vi "readFromXML.vi"(8 "error in (no error)":errorcluster, 10 "XML in":string, 11 "WSSet in":refnum<class "WSSet.lvclass">) -> (0 "error out":errorcluster, 3 "WSSet out":refnum<class "WSSet.lvclass">)   [LabVIEW 2014, in "TCSDataDefinitions.lvlib" / "TCSWeatherServerCommand.lvlib" / "WSSet.lvclass"]
uses:
  WSSet.lvclass
  <userlib>/Common/UnitsAndXML/FlattenItemWithUnitToXML/FlattenPressureToXML/PressureUnit.ctl
  <userlib>/Common/UnitsAndXML/FlattenItemWithUnitToXML/FlattenTemperatureAbsToXML/TemperatureAbsUnit.ctl
  WSSet.lvclass/WSSet.ctl
  TCSWeatherServerCommand/TCSWeatherServerCommand.lvclass
  <userlib>/Common/UnitsAndXML/UnitsAndXML.lvlib
  <userlib>/Common/XML/XMLParser/XMLParser.lvclass
panel:
  out "relativeHumidity_percent":dbl
  out "temperature_degC":dbl[unit]=273.15
  out "pressure_mbar":dbl[unit]
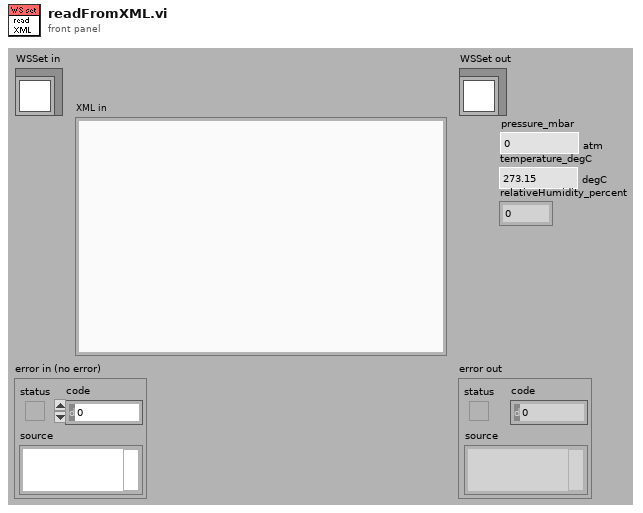
[diagram p1: front panel]
types:
  T1 = typedef "UnitsAndXML.lvlib/TemperatureAbsUnit.ctl" = enum16{"K", "degC", "degF"}
  T2 = typedef "UnitsAndXML.lvlib/PressureUnit.ctl" = enum16{"Pa", "atm", "bar", "mbar", "m.Hg", "psi", "torr"}
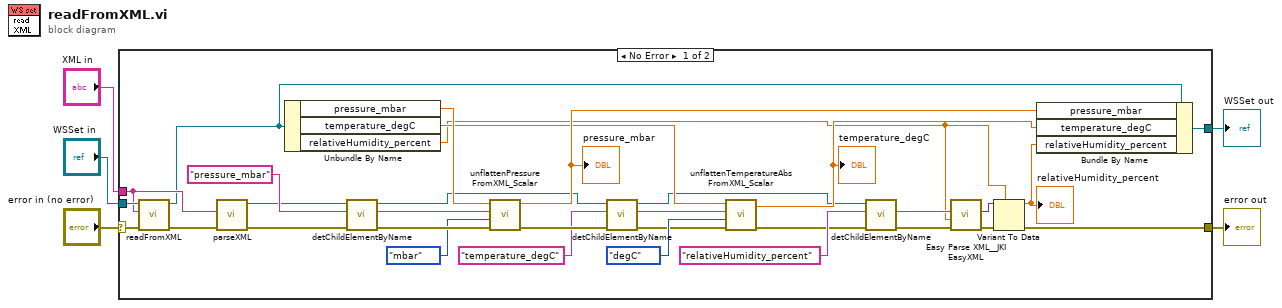
[diagram p0: block diagram]
diagram:
  n1 = case shown="No Error" "error in (no error)" {
    selector: "error in (no error)" -> [w33 w39]
    tunnel: [w9 w39] -> w4
    tunnel: [w30 w38] -> w2
    tunnel: "WSSet in" -> [w35 w38]
    tunnel: "XML in" -> [w34 _]
    frame No Error {
      n2 = call-parent "readFromXML.vi"("error in (no error)"=w33, "XML in"=w34, "TCSWeatherServerCommand in"=w35) -> ("error out"=w32:errorcluster, "TCSWeatherServerCommand out"=w31:refnum<class "WSSet.lvclass">)  [unwired: 7 out]
      n3 = call <userlib>:"parseXML.vi"("error in (no error)"=w32, "XMLString in"=w34) -> ("error out"=w36:errorcluster, "Element out"=w8:refnum<class "XMLParser.lvclass">)  [unwired: 8 in]
      n4 = Unbundle By Name(w31) -> ("pressure_mbar"=w29:dbl[unit], "temperature_degC"=w23:dbl[unit], "relativeHumidity_percent"=w12:dbl)
      n5 = call <userlib>:"detChildElementByName.vi"("error in (no error)"=w36, "childName"="pressure_mbar" ("ChildName"), "Element in"=w8) -> ("error out"=w27:errorcluster, "childXML"=w28:string, "Element out"=w7:refnum<class "XMLParser.lvclass">)  [unwired: 5 in, 1 out]
      n6 = call <userlib>:"unflattenPressureFromXML_Scalar.vi"("error in (no error)"=w27, "pressureUnitInXML"=PressureUnit."mbar", "xmlString"=w28, "pressureForType"=w29) -> ("error out"=w25:errorcluster, "pressure"=w24:dbl[unit])  [unwired: 6 in]
      "pressure_mbar" <- w24
      n7 = call <userlib>:"detChildElementByName.vi"("error in (no error)"=w25, "childName"="temperature_degC" ("ChildName"), "Element in"=w7) -> ("error out"=w18:errorcluster, "childXML"=w22:string, "Element out"=w6:refnum<class "XMLParser.lvclass">)  [unwired: 5 in, 1 out]
      n8 = call <userlib>:"unflattenTemperatureAbsFromXML_Scalar.vi"("error in (no error)"=w18, "temperatureAbsUnitInXML"=TemperatureAbsUnit."degC", "xmlString"=w22, "temperatureAbsForType"=w23) -> ("error out"=w17:errorcluster, "temperatureAbs"=w16:dbl[unit])  [unwired: 6 in]
      "temperature_degC" <- w16
      n9 = call <userlib>:"detChildElementByName.vi"("error in (no error)"=w17, "childName"="relativeHumidity_percent" ("ChildName"), "Element in"=w6) -> ("error out"=w10:errorcluster, "childXML"=w15:string)  [unwired: 5 in, 2 out]
      n10 = call <vilib>:"Easy Parse XML__JKI EasyXML.vi"("error in (no error)"=w10, "LabVIEW Data (Type)"=w12, "XML String"=w15) -> ("error out"=w14:errorcluster, "LabVIEW Data"=w13:variant)  [unwired: 7 in]
      n11 = Variant To Data(error in=w14, type=w12, Variant=w13) -> (data=w11:dbl, error out=w9:errorcluster)
      "relativeHumidity_percent" <- w11
      n12 = Bundle By Name(cluster=w31, "pressure_mbar"=w24, "temperature_degC"=w16, "relativeHumidity_percent"=w11) -> (w30:refnum<class "WSSet.lvclass">)
    }
    frame Error {
    }
  }
  "error out" <- w4
  "WSSet out" <- w2
